vi "Nm_to_A.vi"(11 "Torque [Nm]":dbl) -> (3 "Current [A]":dbl)   [LabVIEW 2019]
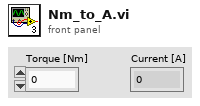
[diagram p1: front panel]
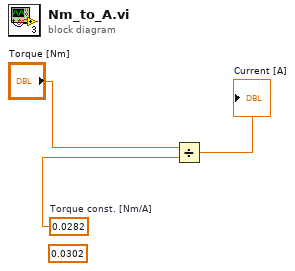
[diagram p0: block diagram]
diagram:
  (unwired) 0.0302
  w2 = 0.0282  # Torque const. [Nm/A]
  n1 = Divide(x="Torque [Nm]", y=w2) -> (x/y=→"Current [A]":dbl)
